vi "getWFMQueue.vi"(8 "error in (no error)":errorcluster, 10 "wait for min buffer?":bool, 11 "DAQmx in":refnum<class "DAQmx.lvclass">) -> (0 "error out":errorcluster, 1 "timed out?":bool, 3 "DAQmx out":refnum<class "DAQmx.lvclass">)   [LabVIEW 2019, in "DAQmx.lvclass"]
uses:
  DAQmx.lvclass
  DAQmx.lvclass/DAQmx.ctl
  <vilib>/Utility/error.llb/Error Cluster From Error Code.vi
  <vilib>/ErrorRing/Error Ring.xnode
panel:
  out "AO Queue Refnum":i32
  out "v timed out":bool
  out "AO queue #":i32
  out "Y /empty":bool
  out "X /empty":bool
  out "AO /empty":bool
  out "^ /empty":bool
  out "time waiting for buffer":dbl format="%#_6p"
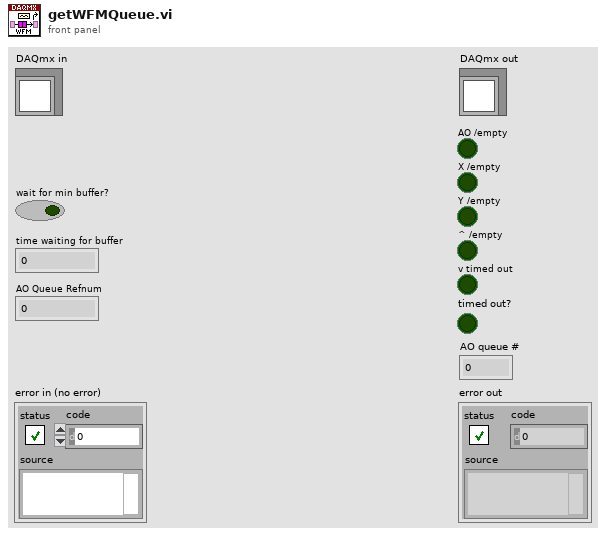
[diagram p1: front panel]
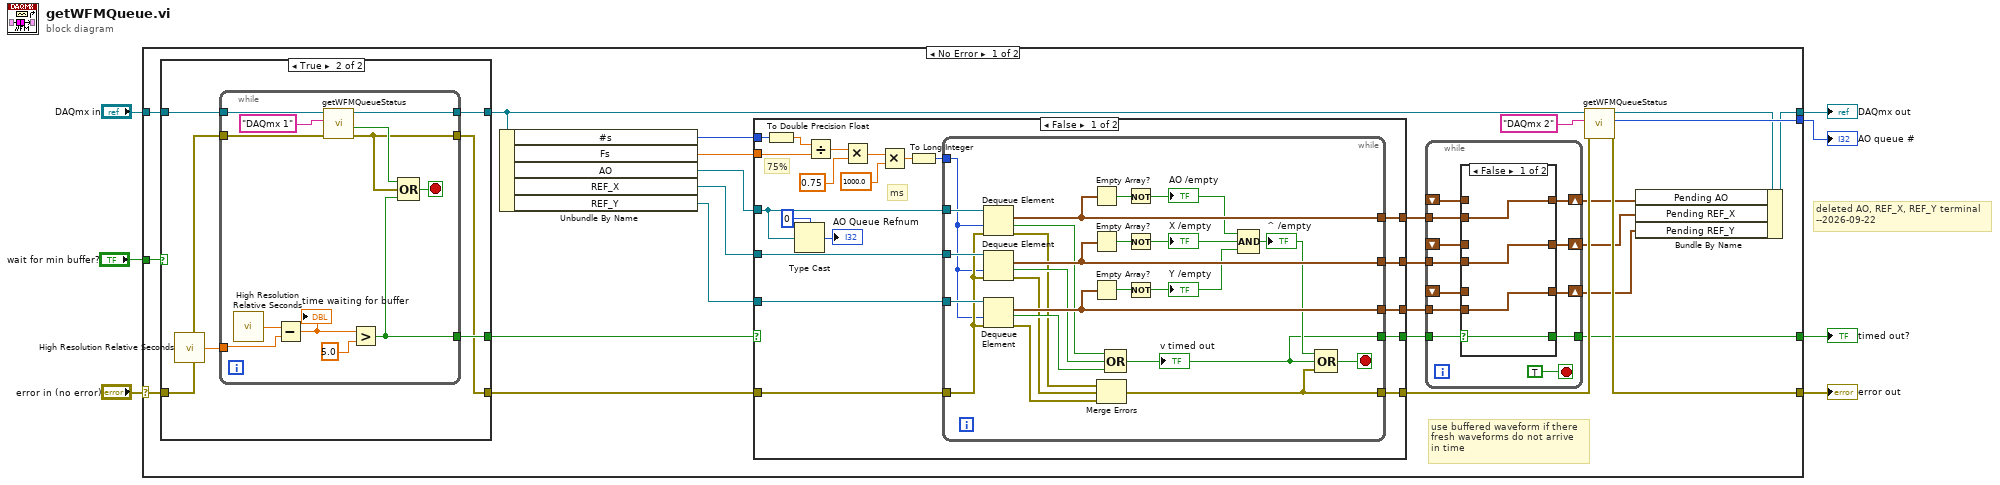
[diagram p0: block diagram]
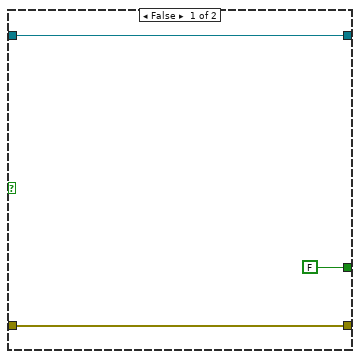
[diagram p2: hidden frame]
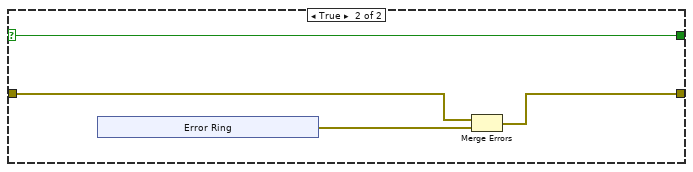
[diagram p3: hidden frame]
diagram:
  # "deleted AO, REF_X, REF_Y terminal\n--2026-09-22"
  n1 = case shown="No Error" "error in (no error)" {
    selector: "error in (no error)" -> [w28 w127]
    tunnel: [w22 w127] -> w3
    tunnel: [w8 w126] -> w1
    tunnel: "DAQmx in" -> [w30 w126]
    tunnel: [w15 _] -> w5
    tunnel: "wait for min buffer?" -> [w26 _]
    tunnel: [w20 _] -> w2
    frame No Error {
      # "use buffered waveform if there\nfresh waveforms do not arrive\nin time"
      n2 = case shown="True" w26 {
        tunnel: [w33 w41] -> w24
        tunnel: w30 -> [w33 w40]
        tunnel: [FALSE w39] -> w29
        tunnel: w28 -> [w34 w38]
        tunnel: [w34 w37] -> w27
        frame False {
        }
        frame True {
          n3 = call <vilib>:"High Resolution Relative Seconds.vi"() -> ("relative seconds"=w36:dbl)
          n4 = while {
            tunnel: w36 -> [w43]
            tunnel: [w48] -> w39
            tunnel: w38 -> [w47]
            tunnel: [w46] -> w37
            tunnel: w40 -> [w52]
            tunnel: [w53] -> w41
            stop <- w49 stop-if-true
            n5 = call <vilib>:"High Resolution Relative Seconds.vi"() -> ("relative seconds"=w44:dbl)
            n6 = Subtract(x=w44, y=w43) -> (x-y=w42:dbl)
            "time waiting for buffer" <- w42
            n7 = call "getWFMQueueStatus.vi"("error in (no error)"=w47, "instance"="DAQmx 1", "DAQmx in"=w52) -> ("error out"=w46:errorcluster, "Min AO Queue Filled"=w50:bool, "DAQmx out"=w53:refnum<class "DAQmx.lvclass">)  [unwired: 5 in, 1 out]
            n8 = Greater?(x=w42, y=5.0) -> (0:w48:bool)
            n9 = Compound Arithmetic op=OR(w50, w46, w48) -> (w49:bool)
          }
        }
      }
      n10 = Unbundle By Name(w24) -> ("#s"=w14:i32, "Fs"=w21:dbl, "AO"=w13:refnum<queue>, "REF_X"=w31:refnum<queue>, "REF_Y"=w32:refnum<queue>)
      n11 = case shown="False" w29 {
        selector: w29 -> [_ w98]
        tunnel: [w73 w98] -> w18
        tunnel: [w72 w100] -> w23
        tunnel: [w71 _] -> w19
        tunnel: [w70 _] -> w17
        tunnel: [w69 _] -> w16
        tunnel: w13 -> [w56 _]
        tunnel: w31 -> [w68 _]
        tunnel: w32 -> [w67 _]
        tunnel: w27 -> [w66 w99]
        tunnel: w21 -> [w64 _]
        tunnel: w14 -> [w61 _]
        frame False {
          # "ms"
          # "75%"
          n12 = To Double Precision Float(number=w61) -> (double precision float=w60:dbl)
          n13 = Type Cast(type=0, x=w56) -> (*(type *) &x=→"AO Queue Refnum":i32)
          n14 = Divide(x=w60, y=w64) -> (x/y=w65:dbl)
          n15 = Multiply(x=w65, y=0.75 ("timeout in ms (-1)")) -> (x*y=w59:dbl)
          n16 = Multiply(x=w59, y=1000.0 ("timeout in ms (-1)")) -> (x*y=w58:dbl)
          n17 = To Long Integer(number=w58) -> (32bit integer=w62:i32)
          n18 = while {
            tunnel: [w74] -> w73
            tunnel: [w79] -> w72
            tunnel: w56 -> [w97]
            tunnel: w68 -> [w96]
            tunnel: w67 -> [w95]
            tunnel: [w84] -> w71
            tunnel: [w85] -> w70
            tunnel: [w94] -> w69
            tunnel: w66 -> [w86]
            tunnel: w62 -> [w83]
            stop <- w90 stop-if-true
            n19 = Dequeue Element(queue=w97, timeout in ms (-1)=w83, error in (no error)=w86) -> (element=w84:waveform(dbl)[], timed out?=w82:bool, error out=w80:errorcluster)  [unwired: 1 out]
            n20 = Dequeue Element(queue=w96, timeout in ms (-1)=w83, error in (no error)=w86) -> (element=w85:waveform(dbl)[], timed out?=w89:bool, error out=w87:errorcluster)  [unwired: 1 out]
            n21 = Dequeue Element(queue=w95, timeout in ms (-1)=w83, error in (no error)=w86) -> (element=w94:waveform(dbl)[], timed out?=w88:bool, error out=w81:errorcluster)  [unwired: 1 out]
            n22 = Empty Array?(array=w84) -> (empty?=w93:bool)
            n23 = Empty Array?(array=w85) -> (empty?=w92:bool)
            n24 = Empty Array?(array=w94) -> (empty?=w91:bool)
            n25 = Merge Errors(w80, w87, w81) -> (w79:errorcluster)
            n26 = Compound Arithmetic op=OR(w82, w89, w88) -> (w74:bool)
            "v timed out" <- w74
            n27 = Not(x=w93) -> (.not. x?=w75:bool)
            "AO /empty" <- w75
            n28 = Not(x=w92) -> (.not. x?=w77:bool)
            "X /empty" <- w77
            n29 = Not(x=w91) -> (.not. x?=w76:bool)
            "Y /empty" <- w76
            n30 = Compound Arithmetic op=AND(w75, w77, w76) -> (w78:bool)
            "^ /empty" <- w78
            n31 = Compound Arithmetic op=OR(w78, w74, w79) -> (w90:bool)
          }
        }
        frame True {
          n32 = xnode "Error Ring"() -> ("error out"=w101:errorcluster)
          n33 = Merge Errors(w99, w101) -> (w100:errorcluster)
        }
      }
      n34 = while {
        tunnel: w19 -> [w114]
        shift-right: [w115] -> w12
        shift-left: _ -> [w107]
        tunnel: w18 -> [w116]
        tunnel: w17 -> [w112]
        shift-right: [w113] -> w11
        shift-left: _ -> [w108]
        tunnel: w16 -> [w110]
        shift-right: [w111] -> w10
        shift-left: _ -> [w109]
        tunnel: [w106] -> w15
        stop <- TRUE stop-if-true
        n35 = case shown="False" w116 {
          selector: w116 -> [w118 w122]
          tunnel: [w121 w123] -> w115
          tunnel: w114 -> [w121 _]
          tunnel: [w120 w124] -> w113
          tunnel: w112 -> [w120 _]
          tunnel: [w119 w125] -> w111
          tunnel: w110 -> [w119 _]
          tunnel: w109 -> [_ w125]
          tunnel: w108 -> [_ w124]
          tunnel: w107 -> [_ w123]
          tunnel: [w118 w122] -> w106
          frame False {
          }
          frame True {
          }
        }
      }
      n36 = call "getWFMQueueStatus.vi"("error in (no error)"=w23, "instance"="DAQmx 2", "DAQmx in"=w24) -> ("error out"=w22:errorcluster, "AO queue #"=w20:i32, "DAQmx out"=w9:refnum<class "DAQmx.lvclass">)  [unwired: 5 in, 1 out]
      n37 = Bundle By Name(cluster=w9, "Pending AO"=w12, "Pending REF_X"=w11, "Pending REF_Y"=w10) -> (w8:refnum<class "DAQmx.lvclass">)
    }
    frame Error {
    }
  }
  "error out" <- w3
  "DAQmx out" <- w1
  "timed out?" <- w5
  "AO queue #" <- w2
